vi "just_move.vi"(2 "mm":dbl, 3 "Motor":u16(ring) items=["X", "Y", "Z", "Gluer", "Spint"]) -> (0 "output":string, 1 "command":string)   [LabVIEW 2015]
panel:
  in  "Reset Program":bool
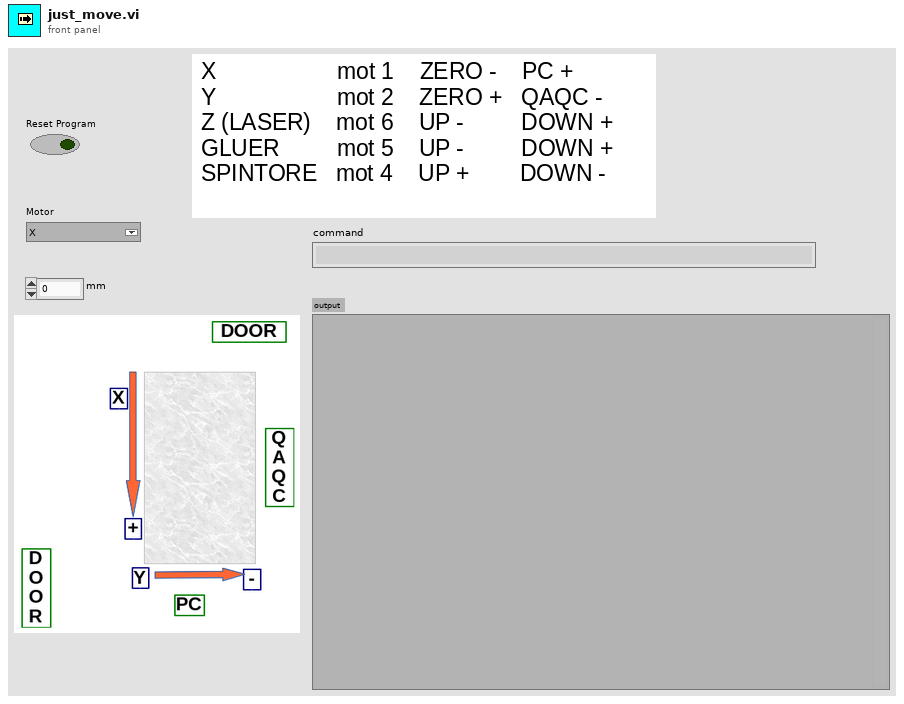
[diagram p1: front panel]
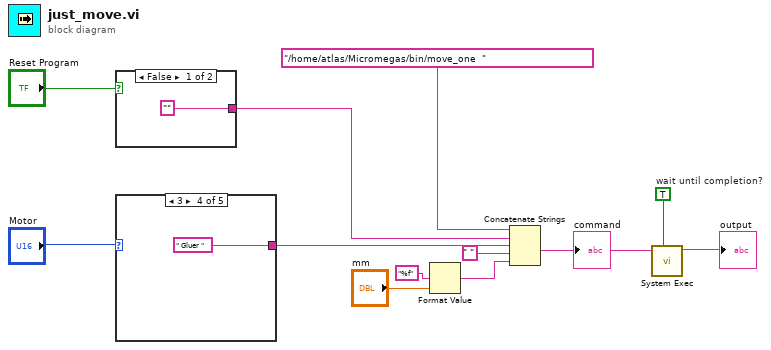
[diagram p0: block diagram]
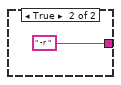
[diagram p2: hidden frame]
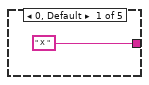
[diagram p3: hidden frame]
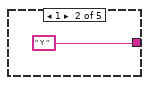
[diagram p4: hidden frame]
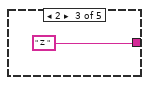
[diagram p5: hidden frame]
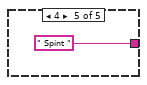
[diagram p6: hidden frame]
diagram:
  w12 = TRUE  # wait until completion?
  n1 = case shown="False" "Reset Program" {
    tunnel: ["" " -r "] -> w4
    frame False {
    }
    frame True {
    }
  }
  n2 = case shown="3" "Motor" {
    tunnel: [" X " ("motore") " Y " ("motore") " Z " ("motore") " Gluer " ("motore") " Spint " ("motore")] -> w7
    frame 0, Default {
    }
    frame 1 {
    }
    frame 2 {
    }
    frame 3 {
    }
    frame 4 {
    }
  }
  n3 = Format Value(format string="%f", value (0)="mm") -> (output string=w1:string)  [unwired: 1 in]
  n4 = Concatenate Strings("/home/atlas/Micromegas/bin/move_one  " ("string"), w4, w7, " " ("string"), w1) -> (w10:string)
  "command" <- w10
  n5 = call <vilib>:"System Exec.vi"("wait until completion? (T)"=w12, "command line"=w10) -> ("standard output"=→"output":string)  [unwired: 6 in, 3 out]
